vi "计时.vi"() -> ()   [LabVIEW 2010]
panel:
  out "消耗时间":u32
  out "循环次数":i32
  out "当前累积数":dbl
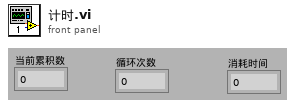
[diagram p1: front panel]
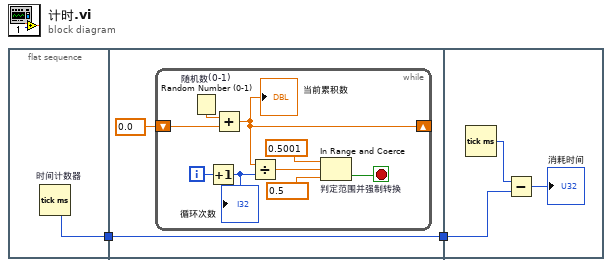
[diagram p0: block diagram]
diagram:
  n1 = flat-sequence {
    tunnel: [w3] -> w2
    tunnel: w2 -> [w4]
    tunnel: [w4] -> w1
    tunnel: w1 -> [w16]
    frame #0 {
      n2 = Tick Count (ms) "时间计数器"() -> (millisecond timer value=w3:u32)
    }
    frame #1 {
      n3 = while {
        shift-right: [w10] -> _
        shift-left: 0.0 -> [w13]
        i -> [w12]
        stop <- w8 stop-if-true
        n4 = Random Number (0-1) "随机数(0-1)"() -> (number: 0 to 1=w14:dbl)
        n5 = Increment(x=w12) -> (x+1=w11:i32)
        "循环次数" <- w11
        n6 = Add(x=w14, y=w13) -> (x+y=w10:dbl)
        "当前累积数" <- w10
        n7 = Divide(x=w10, y=w11) -> (x/y=w9:dbl)
        n8 = In Range and Coerce "判定范围并强制转换"(upper limit=0.5001, x=w9, lower limit=0.5) -> (In Range?=w8:bool)  [unwired: 1 out]
      }
    }
    frame #2 {
      n9 = Tick Count (ms)() -> (millisecond timer value=w17:u32)
      n10 = Subtract(x=w17, y=w16) -> (x-y=→"消耗时间":u32)
    }
  }
